vi "KE2260B Read Output.vi"(8 "error in (no error)":errorcluster, 11 "VISA resource name":refnum<visa-resource-name>) -> (0 "error out":errorcluster, 1 "Actual Current Level (A)":dbl format="%.3g", 2 "Actual Voltage Level (V)":dbl format="%.3g", 3 "VISA resource name out":refnum<visa-resource-name>)   [LabVIEW 2016, in "Keithley 2260B.lvlib"]
doc: "Returns the actual voltage level and actual current level."
uses:
  Keithley 2260B.lvlib
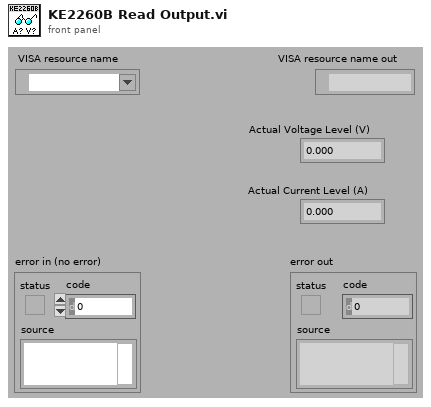
[diagram p1: front panel]
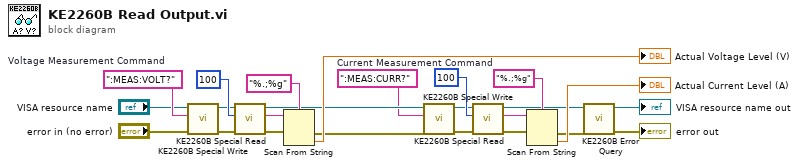
[diagram p0: block diagram]
diagram:
  w5 = ":MEAS:CURR?"  # Current Measurement Command
  w11 = ":MEAS:VOLT?"  # Voltage Measurement Command
  n1 = call "KE2260B Special Write.vi"("error in (no error)"="error in (no error)", "Write Buffer (\"\")"=w11, "VISA session"="VISA resource name") -> ("error out"=w13:errorcluster, "dup VISA session"=w12:refnum<visa-resource-name>)  [unwired: 6 in, 1 out]
  n2 = call "KE2260B Special Read.vi"("error in (no error)"=w13, "byte count"=u32 100, "VISA session"=w12) -> ("error out"=w4:errorcluster, "read buffer"=w20:string, "dup VISA session"=w6:refnum<visa-resource-name>)  [unwired: 5 in, 1 out]
  n3 = Scan From String(format string="%.;%g", input string=w20, error in=w4) -> (error out=w3:errorcluster, output 1=→"Actual Voltage Level (V)":dbl)  [unwired: 2 in, 2 out]
  n4 = call "KE2260B Special Write.vi"("error in (no error)"=w3, "Write Buffer (\"\")"=w5, "VISA session"=w6) -> ("error out"=w8:errorcluster, "dup VISA session"=w7:refnum<visa-resource-name>)  [unwired: 6 in, 1 out]
  n5 = call "KE2260B Special Read.vi"("error in (no error)"=w8, "byte count"=u32 100, "VISA session"=w7) -> ("error out"=w2:errorcluster, "read buffer"=w17:string, "dup VISA session"=w14:refnum<visa-resource-name>)  [unwired: 5 in, 1 out]
  n6 = Scan From String(format string="%.;%g", input string=w17, error in=w2) -> (error out=w1:errorcluster, output 1=→"Actual Current Level (A)":dbl)  [unwired: 2 in, 2 out]
  n7 = call "KE2260B Error Query.vi"("error in (no error)"=w1, "VISA resource name"=w14) -> ("error out"=→"error out":errorcluster, "VISA resource name out"=→"VISA resource name out":refnum<visa-resource-name>)  [unwired: 6 in, 2 out]
